vi "Send data_to_parser.vi"(5 "port":u16, 6 "connection ID out":refnum<k16>, 7 "Message Priority (Normal)":T1=enum."Normal", 8 "error in (no error)":errorcluster, 9 "address":u32, 10 "udp message":string, 11 "Message Enqueuer":refnum<class "Message Enqueuer.lvclass">) -> (0 "error out":errorcluster, 3 "Message Enqueuer out":refnum<class "Message Enqueuer.lvclass">)   [LabVIEW 2025, in "UDP_receiver.lvlib" / "data_to_parser Msg.lvclass"]
doc: "This VI sends the message to an actor."
uses:
  data_to_parser Msg.lvclass
  <vilib>/ActorFramework/Message Enqueuer/Message Enqueuer.lvclass
  <vilib>/ActorFramework/Message Enqueuer/Message Priority.ctl
  Applications/National Instruments/LabVIEW 2025 64-bit/vi.lib/ActorFramework/Message/Message.lvclass
  data_to_parser Msg.lvclass/data_to_parser Msg.ctl
  <vilib>/ActorFramework/Message Enqueuer/Message Enqueuer.lvclass/Message Enqueuer.ctl
  <vilib>/ActorFramework/Message Priority Queue/Priority Enqueue.vi
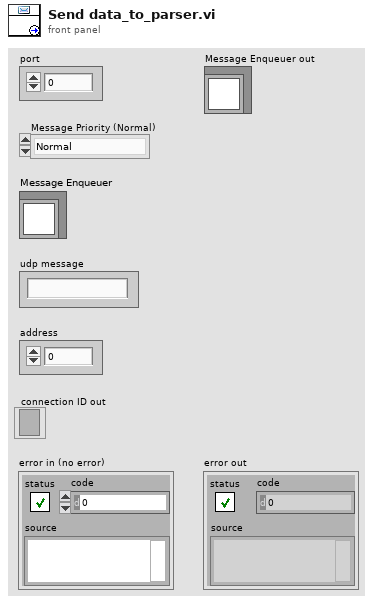
[diagram p1: front panel]
types:
  T1 = typedef "Actor Framework.lvlib/Message Enqueuer.lvclass/Message Priority.ctl" = enum16{"Low", "Normal", "High"}
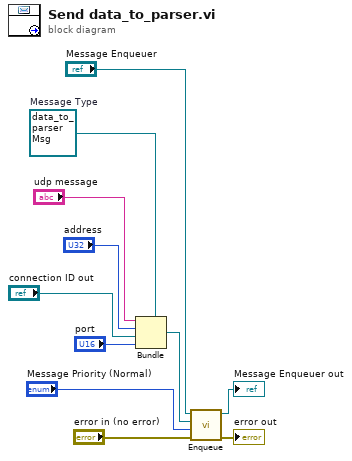
[diagram p0: block diagram]
diagram:
  w8 = refnum<class "data_to_parser Msg.lvclass"> refnum  # Message Type
  n1 = Bundle(cluster=w8, "udp message", "address", "connection ID out", "port") -> (w7:refnum<class "data_to_parser Msg.lvclass">)
  n2 = call <vilib>:"Enqueue.vi"("error in (no error)"="error in (no error)", "Message Priority (Normal)"="Message Priority (Normal)", "Message"=w7, "Message Enqueuer in"="Message Enqueuer") -> ("error out"=→"error out":errorcluster, "Message Enqueuer out"=→"Message Enqueuer out":refnum<class "Message Enqueuer.lvclass">)  [unwired: 6 in]
